vi "Blob_Probe.vi"(11 "Blob":refnum<class "Blob.lvclass">) -> (2 "Value String":string, 3 "Pause VI":bool)   [LabVIEW 2020, in "OpenLvVision_OpenCv.lvlib" / "Blob.lvclass"]
uses:
  Blob.lvclass
  C:/Users/lukas/Downloads/OpenLvVision_OpenCv/SourceCode/LabView/OpenLvVision_OpenCv/_LvHelpers/EdvrObject/EdvrObject.lvclass
  TypeDef/BlobInfo.ctl
  TypeDef/NchwType.ctl
  _LvHelpers/EdvrObject/EdvrObject.lvclass/EdvrObject.ctl
  _LvHelpers/EdvrObject/EdvrObject.lvclass
  OpenLvVision_OpenCv.lvlib
panel:
  out "BlobInfo":T1
  out "Reference":u64 format="%.0x"
  out "NCHW Blob":sgl[][][][](array[numeric])
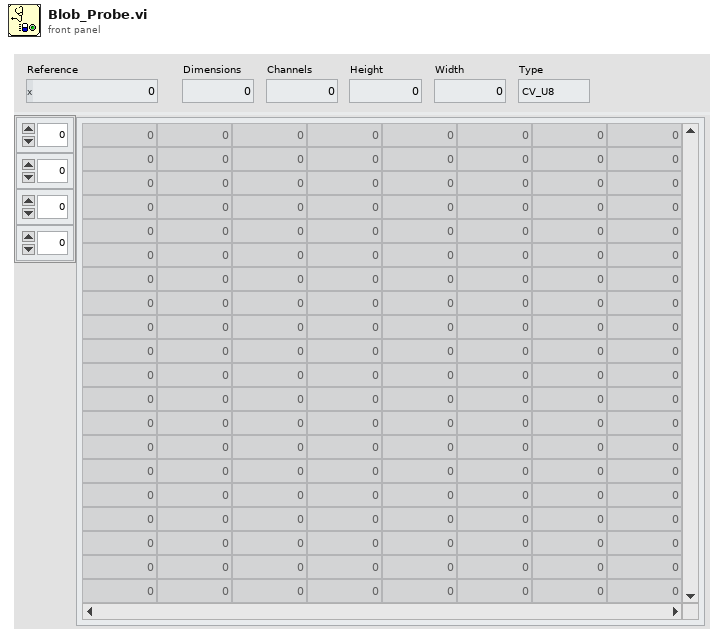
[diagram p1: front panel]
types:
  T1 = typedef "OpenLvVision_OpenCv.lvlib/BlobInfo.ctl" = cluster{"Dimensions":i32, "Channels":i32, "Height":i32, "Width":i32, "Type":T2}
  T2 = typedef "OpenLvVision_OpenCv.lvlib/NchwType.ctl" = enum16{"CV_U8", "CV_8S", "CV_16U", "CV_16S", "CV_32S", "CV_32F", "CV_64F", "CV_16F"}
  T3 = typedef "OpenLvVision_OpenCv.lvlib/EdvrObject.lvclass/Edvr.ctl" = refnum<data-value>
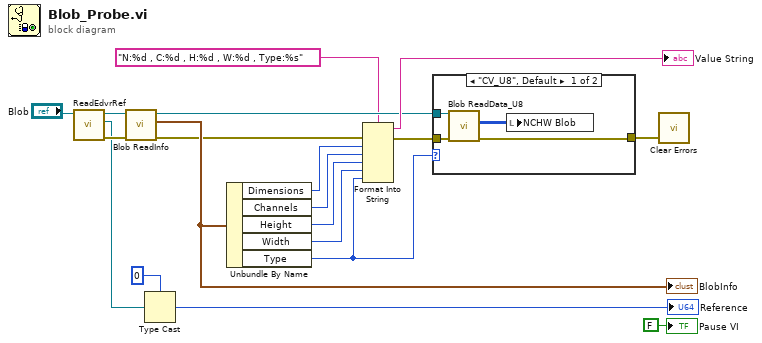
[diagram p0: block diagram]
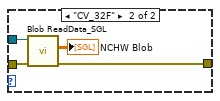
[diagram p2: hidden frame]
diagram:
  n1 = call "ReadEdvrRef.vi"("EdvrObject in"="Blob") -> ("error out"=w14:errorcluster, "Edvr"=w13:T3, "EdvrObject out"=w15:refnum<class "Blob.lvclass">)  [unwired: 8 in]
  n2 = call "Blob ReadInfo.vi"("error in (no error)"=w14, "Blob in"=w15) -> ("error out"=w11:errorcluster, "BlobInfo"=w12:T1, "Blob out"=w4:refnum<class "Blob.lvclass">)  [unwired: 7 in]
  "BlobInfo" <- w12
  n3 = Type Cast(type=u64 0, x=w13) -> (*(type *) &x=→"Reference":u64)
  n4 = Unbundle By Name(w12) -> ("Dimensions"=w10:i32, "Channels"=w9:i32, "Height"=w8:i32, "Width"=w7:i32, "Type"=w1:T2)
  n5 = Format Into String(format string="N:%d , C:%d , H:%d , W:%d , Type:%s", error in=w11, w10, w9, w8, w7, w1) -> (resulting string=→"Value String":string, error out=w5:errorcluster)  [unwired: 1 in]
  n6 = case shown="\"CV_U8\", Default" w1 {
    tunnel: w5 -> [w22 w26]
    tunnel: w4 -> [w23 w27]
    tunnel: [w21 w25] -> w2
    frame "CV_U8", Default {
      n7 = call "Blob ReadData_U8.vi"("error in (no error)"=w22, "Blob in"=w23) -> ("error out"=w21:errorcluster, "NCHW Blob"=w20:u8[][][][])  [unwired: 7 in, 1 out]
      n8 = local write "NCHW Blob"(w20) -> ()
    }
    frame "CV_32F" {
      n9 = call "Blob ReadData_SGL.vi"("error in (no error)"=w26, "Blob in"=w27) -> ("error out"=w25:errorcluster, "NCHW Blob"=→"NCHW Blob":sgl[][][][])  [unwired: 7 in, 1 out]
    }
  }
  n10 = call <vilib>:"Clear Errors.vi"("error in (no error)"=w2) -> ()  [unwired: 5 in, 2 out]
  "Pause VI" <- FALSE
